vi "tstp_can_request_and_get_response.vi"(10 "簇":T1, 11 "路径输入":path) -> (2 "返回类型":i32, 3 "路径输出":path)   [LabVIEW 2019]
panel:
  out "诊断应答":u8[](array[numeric])
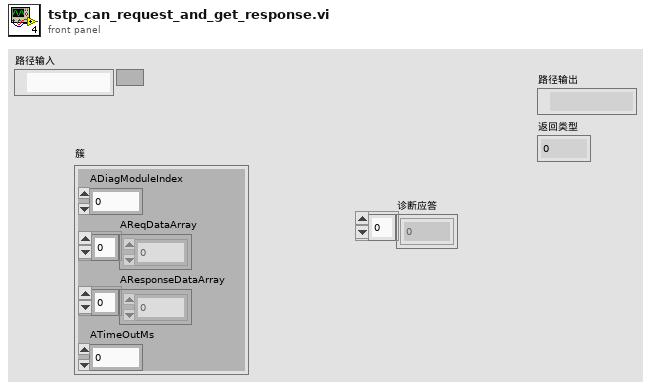
[diagram p1: front panel]
types:
  T1 = cluster{"ADiagModuleIndex":i32, "AReqDataArray":u8[], "AResponseDataArray":u8[], "ATimeOutMs":i32}
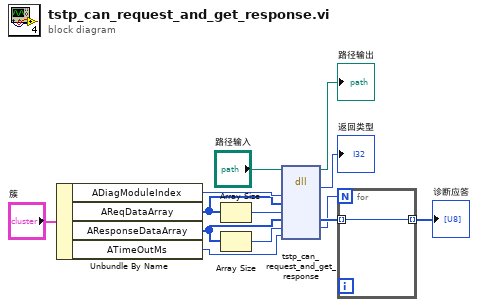
[diagram p0: block diagram]
diagram:
  n1 = Unbundle By Name("簇") -> ("ADiagModuleIndex"=w9:i32, "AReqDataArray"=w6:u8[], "AResponseDataArray"=w2:u8[], "ATimeOutMs"=w8:i32)
  n2 = Array Size(array=w6) -> (size(s)=w7:i32)
  n3 = Array Size(array=w2) -> (size(s)=w1:i32)
  n4 = dll-call lib="C:/Users/XYY/Desktop/LabView Demo/TSCAN_LB2018_V1.3_20220301/Config/TSMaster.dll" fn="tstp_can_request_and_get_response"(path in="路径输入", "ADiagModuleIndex"=w9, "AReqDataArray"=w6, "AReqDataSize"=w7, "AResponseDataArray"=w2, "AResponseDataSize"=w1, "ATimeOutMs"=w8) -> (path out=→"路径输出":path, "返回类型"=→"返回类型":i32, "AResponseDataArray"=w5:u8[], "AResponseDataSize"=w4:i32)  [unwired: 6 in, 1 out]
  n5 = for {
    N: w4 -> [_]
    tunnel: w5 -> [w14] mode=indexing
    tunnel: [w14] -> w3 mode=indexing
  }
  "诊断应答" <- w3
